vi "SetStagePosition.vi"(0 "DemoCamera in":refnum<class "DemoCamera.lvclass">, 5 "Label":string, 7 "AbsPosition?":bool=TRUE, 9 "Value":dbl format="%#_13g", 11 "error in (no error)":errorcluster) -> (4 "DemoCamera out":refnum<class "DemoCamera.lvclass">, 15 "error out":errorcluster)   [LabVIEW 2020, in "DemoCamera.lvlib" / "DemoCamera.lvclass"]
uses:
  DemoCamera.lvclass
  C:/Program Files/National Instruments/LabVIEW 2020/vi.lib/ActorFramework/Actor/Actor.lvclass
  <vilib>/ActorFramework/Actor/Actor.lvclass/Actor.ctl
  Interface/StageController Messages/SetStagePosition Msg/SetStagePosition Msg.lvclass/SetStagePosition Msg.ctl
  <vilib>/ActorFramework/Message Enqueuer/Message Enqueuer.lvclass/Message Enqueuer.ctl
  <vilib>/ActorFramework/Message Enqueuer/Enqueue.vi
  Interface/StageController Messages/SetStagePosition Msg/SetStagePosition Msg.lvclass
  C:/Program Files/National Instruments/LabVIEW 2020/vi.lib/ActorFramework/Message/Message.lvclass
  <vilib>/ActorFramework/Message Priority Queue/Priority Enqueue.vi
  <vilib>/ActorFramework/Actor/Actor.lvclass
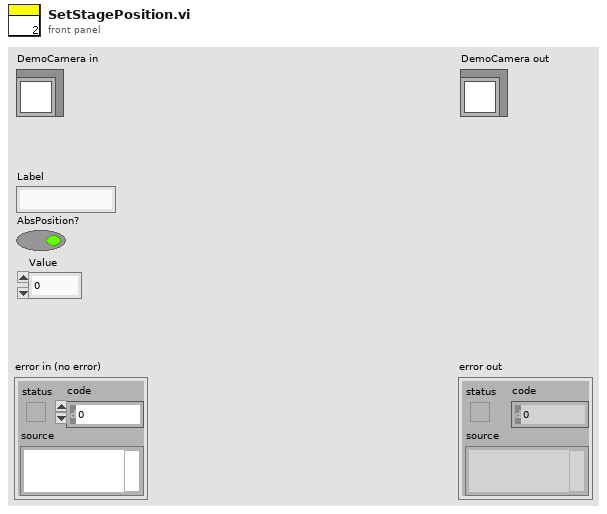
[diagram p1: front panel]
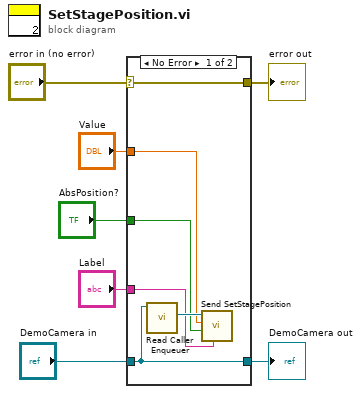
[diagram p0: block diagram]
diagram:
  n1 = case shown="No Error" "error in (no error)" {
    selector: "error in (no error)" -> [w13 w15]
    tunnel: [w13 w15] -> w6
    tunnel: "DemoCamera in" -> [w12 w14]
    tunnel: [w12 w14] -> w4
    tunnel: "Value" -> [w10 _]
    tunnel: "AbsPosition?" -> [w9 _]
    tunnel: "Label" -> [w8 _]
    frame No Error {
      n2 = call <vilib>:"Read Caller Enqueuer.vi"("Actor"=w12) -> ("Caller Enqueuer"=w11:refnum<class "Message Enqueuer.lvclass">)  [unwired: 10 in]
      n3 = call "Send SetStagePosition.vi"("Label"=w8, "AbsPosition?"=w9, "Value"=w10, "Message Enqueuer"=w11) -> ()  [unwired: 6 in, 2 out]
    }
    frame Error {
    }
  }
  "error out" <- w6
  "DemoCamera out" <- w4
